vi "Get LV Strings.vi"(10 "Versions":dbl[](array[numeric])) -> (2 "LabVIEW Strings":string[](array[string]))   [LabVIEW 2013]
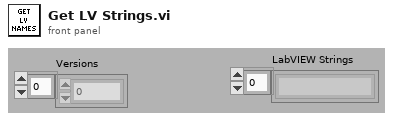
[diagram p1: front panel]
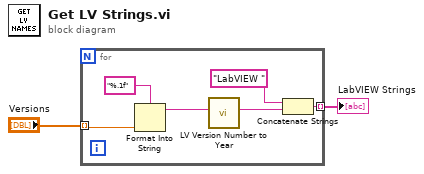
[diagram p0: block diagram]
diagram:
  n1 = for {
    tunnel: "Versions" -> [w8] mode=indexing
    tunnel: [w3] -> w1 mode=indexing
    n2 = Format Into String(format string="%.1f", w8) -> (resulting string=w6:string)  [unwired: 2 in, 1 out]
    n3 = call "LV Version Number to Year.vi"("VI Version"=w6) -> ("LabVIEW Version"=w4:string)  [unwired: 10 in]
    n4 = Concatenate Strings("LabVIEW " ("string"), w4) -> (w3:string)
  }
  "LabVIEW Strings" <- w1
